vi "log analysis_gps.vi"() -> ()   [LabVIEW 2018] (continued)
normal 2 27.000000 0 0\trobot status\t-1.473744\t-2.554606\t9.902600\t-0.433320\t-1.747335\t-47.205490\t0.305000\t0.178000\n\t\n15:53:51.5\tlog_raw\tgps_raw\t#INSPVAXA,USB3,0,49.0,FINESTEERING,2107,284049.550,02008000,471d,15824;INS_ALIGNMENT_COMPLETE,INS_RTKFIXED,37.37010620824,126.72081956922,9.9012,22.3000,-0.1970,0.1771,0.0298,-0.594531132,-1.644459886,132.097505045,0.4329,0.3030,0.5941,0.1170,0.0985,0.0797,0.0945,0.0983,5.1926,0f000001,0*6b710ba0\n\tsystem status\tnormal 2 27.100000 4 0\trobot status\t-1.376142\t-2.662328\t9.901200\t-0.594531\t-1.644460\t-42.097505\t0.274000\t0.222000\n\t\n15:53:52.0\tlog_raw\tgps_raw\t#INSPVAXA,USB3,0,49.0,FINESTEERING,2107,284050.050,02008000,471d,15824;INS_ALIGNMENT_COMPLETE,INS_RTKFIXED,37.37010525413,126.72082070794,9.8986,22.3000,-0.1917,0.2051,-0.0115,-0.516834592,-1.395099600,126.953212153,0.4346,0.3025,0.5938,0.1182,0.0995,0.0796,0.0941,0.0979,5.1828,0f000001,0*22942ac6\n\tsystem status\tnormal 2 27.200000 4 0\trobot status\t-1.275276\t-2.768220\t9.898600\t-0.516835\t-1.395100\t-36.953212\t0.314000\t0.208000\n\t\n15:53:52.5\tlog_raw\tgps_raw\t#INSPVAXA,USB3,0,50.0,FINESTEERING,2107,284050.550,02008000,471d,15824;INS_ALIGNMENT_COMPLETE,INS_RTKFIXED,37.37010440811,126.72082198518,9.8945,22.3000,-0.1594,0.2362,0.0179,-0.435131967,-1.128099811,121.559655858,0.4346,0.3025,0.5938,0.1182,0.0995,0.0796,0.0941,0.0979,5.1828,0f000001,0*78d5de76\n\tsystem status\tnormal 2 27.000000 4 0\trobot status\t-1.162140\t-2.862115\t9.894500\t-0.435132\t-1.128100\t-31.559656\t0.296000\t0.194000\n\t\n15:53:53.0\tlog_raw\tgps_raw\t#DUALANTENNAHEADINGA,USB3,0,50.0,FINESTEERING,2107,284051.000,02008000,d426,15824;INSUFFICIENT_OBS,NONE,-1.000000000,0.000000000,0.000000000,0.0,0.000000000,0.000000000,\"631T\",9,3,3,3,04,00,20,00*f8ed9a8f\n\tsystem status\tnormal 2 27.100000 0 0\trobot status\t-1.053688\t-2.941976\t9.891500\t-0.278851\t-1.155266\t-26.858496\t0.311000\t0.181000\n\t\n15:53:53.5\tlog_raw\tgps_raw\t#INSPVAXA,USB3,0,49.5,FINESTEERING,2107,284051.550,02008000,471d,15824;INS_ALIGNMENT_COMPLETE,INS_RTKFIXED,37.37010293167,126.72082506603,9.8918,22.3000,-0.2006,0.4462,0.0191,-0.487315939,-0.767469623,111.533398827,0.4366,0.3027,0.5935,0.1195,0.1007,0.0795,0.0936,0.0973,5.1774,0f000001,0*2ba22a04\n\tsystem status\tnormal 2 26.900000 0 0\trobot status\t-0.889243\t-3.025977\t9.891800\t-0.487316\t-0.767470\t-21.533399\t0.466000\t0.200000\n\t\n15:53:54.0\tlog_raw\tgps_raw\t\tsystem status\tnormal 2 27.100000 4 0\trobot status\t-0.684813\t-3.109579\t9.890900\t-0.932085\t-0.917029\t-16.735766\t0.443000\t0.242000\n\t\n15:53:54.5\tlog_raw\tgps_raw\t#INSPVAXA,USB3,0,52.0,FINESTEERING,2107,284052.550,02000000,471d,15824;INS_ALIGNMENT_COMPLETE,INS_RTKFIXED,37.37010150239,126.72083015025,9.8922,22.3000,-0.0709,0.4201,0.0154,-1.300322363,-0.251250537,100.734835193,0.4385,0.3032,0.5931,0.1216,0.1015,0.0794,0.0930,0.0966,5.1757,0f000001,0*285f67bd\n\tsystem status\tnormal 2 27.000000 4 0\trobot status\t-0.438892\t-3.184605\t9.892200\t-1.300322\t-0.251251\t-10.734835\t0.551000\t0.120000\n\t\n15:53:55.0\tlog_raw\tgps_raw\t#INSPVAXA,USB3,0,51.0,FINESTEERING,2107,284053.050,02000000,471d,15824;INS_ALIGNMENT_COMPLETE,INS_RTKFIXED,37.37010109323,126.72083278272,9.8918,22.3000,-0.0521,0.4828,-0.0093,-1.553917454,-0.330463200,95.839787961,0.4397,0.3042,0.5928,0.1218,0.1030,0.0794,0.0924,0.0958,5.1723,0f000001,0*925ec3e1\n\tsystem status\tnormal 2 27.000000 4 0\trobot status\t-0.205712\t-3.230016\t9.891800\t-1.553917\t-0.330463\t-5.839788\t0.584000\t0.040000\n\t\n15:53:55.5\tlog_raw\tgps_raw\t#INSPVAXA,USB3,0,51.0,FINESTEERING,2107,284053.550,02000000,471d,15824;INS_ALIGNMENT_COMPLETE,INS_RTKFIXED,37.37010075654,126.72083555357,9.8892,22.3000,-0.0359,0.4357,0.0162,-0.976336983,-0.670873991,90.876153080,0.4397,0.3042,0.5928,0.1218,0.1030,0.0794,0.0924,0.0958,5.1723,0f000001,0*923600d8\n\tsystem status\tnormal 2 27.100000 0 0\trobot status\t0.039726\t-3.267383\t9.889200\t-0.976337\t-0.670874\t-0.876153\t0.520000\t0.127000\n\t\n15:53:56.0\tlog_raw\tgps_raw\t#INSPVAXA,USB3,0,51.0,FINESTEERING,2107,284054.050,02000000,471d,15824;INS_ALIGNMENT_COMPLETE,INS_RTKFIXED,37.37010062155,126.72083812098,9.8896,22.3000,-0.0236,0.4683,-0.0223,-0.929923548,-0.516714504,86.855289806,0.4477,0.3075,0.5936,0.1233,0.1036,0.0794,0.0919,0.0952,5.1660,0f000001,0*98660be2\n\tsystem status\tnormal 2 26.700000 4 0\trobot status\t0.267143\t-3.282365\t9.889600\t-0.929924\t-0.516715\t3.144710\t0.532000\t0.096000\n\t\n15:53:56.5\tlog_raw\tgps_raw\t#INSPVAXA,USB3,0,52.5,FINESTEERING,2107,284054.550,02000000,471d,15824;INS_ALIGNMENT_COMPLETE,INS_RTKFIXED,37.37010072634,126.72084085451,9.8879,22.3000,0.0495,0.4621,-0.0139,-0.890595687,-0.279204622,81.540293866,0.4477,0.3075,0.5936,0.1233,0.1036,0.0794,0.0919,0.0952,5.1660,0f000001,0*57c25e6b\n\tsystem status\tnormal 2 26.800000 4 0\trobot status\t0.509274\t-3.270735\t9.887900\t-0.890596\t-0.279205\t8.459706\t0.455000\t0.258000\n\t\n15:53:57.0\tlog_raw\tgps_raw\t#INSPVAXA,USB3,0,50.5,FINESTEERING,2107,284055.050,02000000,471d,15824;INS_ALIGNMENT_COMPLETE,INS_RTKFIXED,37.37010080652,126.72084262595,9.8861,22.3000,-0.0303,0.1528,0.0096,-0.789228824,0.189504141,79.603141557,0.4534,0.3102,0.5943,0.1271,0.1038,0.0794,0.0915,0.0945,5.1589,0f000001,0*17fda88b\n\tsystem status\texception 2 27.400000 4 160\trobot status\t0.666185\t-3.261836\t9.886100\t-0.789229\t0.189504\t10.396858\t0.260000\t0.206000\n\t\n15:53:57.5\tlog_raw\tgps_raw\t#INSPVAXA,USB3,0,50.5,FINESTEERING,2107,284055.550,02000000,471d,15824;INS_ALIGNMENT_COMPLETE,INS_RTKFIXED,37.37010065353,126.72084269507,9.8843,22.3000,-0.0451,0.0165,0.0094,-0.786160418,0.167323403,79.929360762,0.4534,0.3102,0.5943,0.1271,0.1038,0.0794,0.0915,0.0945,5.1589,0f000001,0*1978198f\n\tsystem status\texception 2 27.700000 0 160\trobot status\t0.672308\t-3.278816\t9.884300\t-0.786160\t0.167323\t10.070639\t0.153000\t0.216000\n\t\n15:53:58.0\tlog_raw\tgps_raw\t#INSPVAXA,USB3,0,50.5,FINESTEERING,2107,284056.050,02000000,471d,15824;INS_ALIGNMENT_COMPLETE,INS_RTKFIXED,37.37010048956,126.72084276872,9.8836,22.3000,-0.0469,0.0143,0.0092,-0.786889601,0.175933665,79.925216666,0.4574,0.3114,0.5945,0.1322,0.1037,0.0794,0.0910,0.0937,5.1545,0f000001,0*13d22f98\n\tsystem status\texception 2 27.700000 0 160\trobot status\t0.678832\t-3.297014\t9.883600\t-0.786890\t0.175934\t10.074783\t0.147000\t0.223000\n\t\n15:53:58.5\tlog_raw\tgps_raw\t#INSPVAXA,USB3,0,51.0,FINESTEERING,2107,284056.550,02000000,471d,15824;INS_ALIGNMENT_COMPLETE,INS_RTKFIXED,37.37010037074,126.72084284514,9.8838,22.3000,-0.0480,0.0175,0.0102,-0.787820604,0.175837290,79.928422775,0.4574,0.3114,0.5945,0.1322,0.1037,0.0794,0.0910,0.0937,5.1545,0f000001,0*7f57341f\n\tsystem status\texception 2 27.700000 0 160\trobot status\t0.685601\t-3.310201\t9.883800\t-0.787821\t0.175837\t10.071577\t0.147000\t0.222000\n\t\n15:53:59.0\tlog_raw\tgps_raw\t#INSPVAXA,USB3,0,51.0,FINESTEERING,2107,284057.050,02000000,471d,15824;INS_ALIGNMENT_COMPLETE,INS_RTKFIXED,37.37010024493,126.72084294147,9.8847,22.3000,-0.0489,0.0209,0.0109,-0.790474431,0.175355820,79.934854744,0.4623,0.3124,0.5946,0.1305,0.1033,0.0793,0.0905,0.0930,5.1443,0f000001,0*1624f0ca\n\tsystem status\texception 2 27.700000 0 160\trobot status\t0.694134\t-3.324164\t9.884700\t-0.790474\t0.175356\t10.065145\t0.147000\t0.222000\n\t\n15:53:59.5\tlog_raw\tgps_raw\t#INSPVAXA,USB3,0,51.0,FINESTEERING,2107,284057.550,02000000,471d,15824;INS_ALIGNMENT_COMPLETE,INS_RTKFIXED,37.37010017546,126.72084302597,9.8865,22.3000,-0.0481,0.0245,0.0114,-0.790674154,0.175795443,79.947588667,0.4623,0.3124,0.5946,0.1305,0.1033,0.0793,0.0905,0.0930,5.1443,0f000001,0*fd60ce92\n\tsystem status\texception 2 27.700000 0 160\trobot status\t0.701619\t-3.331874\t9.886500\t-0.790674\t0.175795\t10.052411\t0.147000\t0.222000\n\t\n15:54:00.0\tlog_raw\tgps_raw\t#INSPVAXA,USB3,0,51.0,FINESTEERING,2107,284058.050,02000000,471d,15824;INS_ALIGNMENT_COMPLETE,INS_RTKFIXED,37.37010009897,126.72084313411,9.8886,22.3000,-0.0478,0.0282,0.0114,-0.793625665,0.175511830,79.961034628,0.4652,0.3130,0.5946,0.1280,0.1027,0.0793,0.0901,0.0925,5.1270,0f000001,0*11f44901\n\tsystem status\tnormal 2 27.700000 0 128\trobot status\t0.711197\t-3.340363\t9.888600\t-0.793626\t0.175512\t10.038965\t0.147000\t0.222000\n\t\n15:54:00.5\tlog_raw\tgps_raw\t#INSPVAXA,USB3,0,52.5,FINESTEERING,2107,284058.550,02000000,471d,15824;INS_ALIGNMENT_COMPLETE,INS_RTKFIXED,37.37010007732,126.72084320054,9.8898,22.3000,-0.0461,0.0304,0.0122,-0.792445810,0.175564347,79.985489957,0.4652,0.3130,0.5946,0.1280,0.1027,0.0793,0.0901,0.0925,5.1270,0f000001,0*ea7ef511\n\tsystem status\texception 2 27.700000 0 160\trobot status\t0.717082\t-3.342766\t9.889800\t-0.792446\t0.175564\t10.014510\t0.147000\t0.222000\n\t\n15:54:01.0\tlog_raw\tgps_raw\t\tsystem status\texception 2 27.700000 0 160\trobot status\t0.724287\t-3.345631\t9.891600\t-0.792125\t0.176872\t9.990955\t0.147000\t0.222000\n\t\n15:54:01.5\tlog_raw\tgps_raw\t#INSPVAXA,USB3,0,48.0,FINESTEERING,2107,284059.550,02000000,471d,15824;INS_ALIGNMENT_COMPLETE,INS_RTKFIXED,37.37010006144,126.72084333190,9.8930,22.3000,-0.0410,0.0333,0.0137,-0.793411742,0.179299471,80.037482880,0.4658,0.3133,0.5945,0.1254,0.1019,0.0793,0.0898,0.0921,5.1054,0f000001,0*b41e64db\n\tsystem status\texception 2 27.700000 0 160\trobot status\t0.728717\t-3.344528\t9.893000\t-0.793412\t0.179299\t9.962517\t0.147000\t0.222000\n\t\n15:54:02.0\tlog_raw\tgps_raw\t#INSPVAXA,USB3,0,48.0,FINESTEERING,2107,284060.050,02000000,471d,15824;INS_ALIGNMENT_COMPLETE,INS_RTKFIXED,37.37010007091,126.72084339799,9.8948,22.3000,-0.0383,0.0348,0.0139,-0.792224776,0.181387989,80.068212083,0.4648,0.3132,0.5944,0.1230,0.1009,0.0793,0.0896,0.0921,5.0831,0f000001,0*0e446c66\n\tsystem status\texception 2 27.700000 0 160\trobot status\t0.734571\t-3.343477\t9.894800\t-0.792225\t0.181388\t9.931788\t0.147000\t0.222000\n\t\n15:54:02.5\tlog_raw\tgps_raw\t#INSPVAXA,USB3,0,51.5,FINESTEERING,2107,284060.550,02000000,471d,15824;INS_ALIGNMENT_COMPLETE,INS_RTKFIXED,37.37010010371,126.72084343010,9.8965,22.3000,-0.0351,0.0351,0.0141,-0.794008331,0.181387588,80.099175193,0.4648,0.3132,0.5944,0.1230,0.1009,0.0793,0.0896,0.0921,5.0831,0f000001,0*6d5ef346\n\tsystem status\texception 2 27.700000 0 160\trobot status\t0.737416\t-3.339837\t9.896500\t-0.794008\t0.181388\t9.900825\t0.147000\t0.222000\n\t\n15:54:03.0\tlog_raw\tgps_raw\t#INSPVAXA,USB3,0,47.0,FINESTEERING,2107,284061.050,02000000,471d,15824;INS_ALIGNMENT_COMPLETE,INS_RTKFIXED,37.37010013657,126.72084347859,9.8982,22.3000,-0.0318,0.0362,0.0140,-0.793134778,0.182296813,80.130371651,0.4625,0.3128,0.5942,0.1207,0.0997,0.0793,0.0895,0.0922,5.0625,0f000001,0*150e9f64\n\tsystem status\texception 2 27.700000 0 160\trobot status\t0.741711\t-3.336190\t9.898200\t-0.793135\t0.182297\t9.869628\t0.147000\t0.222000\n\t\n15:54:03.5\tlog_raw\tgps_raw\t\tsystem status\texception 2 27.700000 0 160\trobot status\t0.745103\t-3.333746\t9.898900\t-0.794686\t0.183659\t9.841140\t0.147000\t0.222000\n\t\n15:54:04.0\tlog_raw\tgps_raw\t#INSPVAXA,USB3,0,47.0,FINESTEERING,2107,284062.050,02000000,471d,15824;INS_ALIGNMENT_COMPLETE,INS_RTKFIXED,37.37010017748,126.72084356719,9.8997,22.3000,-0.0290,0.0363,0.0139,-0.794331592,0.183823168,80.187481896,0.4594,0.3121,0.5941,0.1189,0.0986,0.0793,0.0895,0.0925,5.0451,0f000001,0*0cfca1c0\n\tsystem status\texception 2 27.800000 0 160\trobot status\t0.749559\t-3.331650\t9.899700\t-0.794332\t0.183823\t9.812518\t0.147000\t0.222000\n\t\n15:54:04.5\tlog_raw\tgps_raw\t\tsystem status\texception 2 27.700000 0 160\trobot status\t0.750935\t-3.327984\t9.900000\t-0.792965\t0.186753\t9.783400\t0.147000\t0.222000\n\t\n15:54:05.0\tlog_raw\tgps_raw\t#INSPVAXA,USB3,0,47.5,FINESTEERING,2107,284063.050,02000000,471d,15824;INS_ALIGNMENT_COMPLETE,INS_RTKFIXED,37.37010026095,126.72084358162,9.8989,22.3000,-0.0250,0.0360,0.0144,-0.793980547,0.188879000,80.251853132,0.3252,0.2278,0.4744,0.0459,0.0444,0.0422,0.0723,0.0737,4.9906,0f000005,0*164f8940\n\tsystem status\tnormal 2 27.800000 0 128\trobot status\t0.750837\t-3.322386\t9.898900\t-0.793981\t0.188879\t9.748147\t0.147000\t0.222000\n\t\n15:54:05.5\tlog_raw\tgps_raw\t#INSPVAXA,USB3,0,47.5,FINESTEERING,2107,284063.550,02000000,471d,15824;INS_ALIGNMENT_COMPLETE,INS_RTKFIXED,37.37010060191,126.72084312304,9.8728,22.3000,-0.0145,0.0225,0.0107,-0.798483661,0.197892830,80.372723663,0.3252,0.2278,0.4744,0.0459,0.0444,0.0422,0.0723,0.0737,4.9906,0f000005,0*92bf4382\n\tsystem status\texception 2 27.700000 0 160\trobot status\t0.710217\t-3.284545\t9.872800\t-0.798484\t0.197893\t9.627276\t0.147000\t0.222000\n\t\n15:54:06.0\tlog_raw\tgps_raw\t#INSPVAXA,USB3,0,47.5,FINESTEERING,2107,284064.050,02000000,471d,15824;INS_ALIGNMENT_COMPLETE,INS_RTKFIXED,37.37010092341,126.72084268927,9.8479,22.3000,-0.0050,0.0083,0.0065,-0.802010918,0.203072267,80.489552578,0.3043,0.2119,0.4435,0.0375,0.0370,0.0348,0.0717,0.0735,4.9827,0f000005,0*2a9229fa\n\tsystem status\texception 2 27.700000 0 160\trobot status\t0.671794\t-3.248863\t9.847900\t-0.802011\t0.203072\t9.510447\t0.147000\t0.222000\n\t\n15:54:06.5\tlog_raw\tgps_raw\t#INSPVAXA,USB3,0,52.0,FINESTEERING,2107,284064.550,02000000,471d,15824;INS_ALIGNMENT_COMPLETE,INS_RTKFIXED,37.37010093886,126.72084266042,9.8416,22.3000,-0.0043,0.0064,0.0059,-0.803970150,0.202555305,80.508100729,0.3043,0.2119,0.4435,0.0375,0.0370,0.0348,0.0717,0.0735,4.9827,0f000005,0*b303c02a\n\tsystem status\texception 2 27.800000 0 160\trobot status\t0.669239\t-3.247148\t9.841600\t-0.803970\t0.202555\t9.491899\t0.147000\t0.222000\n\t\n15:54:07.0\tlog_raw\tgps_raw\t#INSPVAXA,USB3,0,48.0,FINESTEERING,2107,284065.050,02000000,471d,15824;INS_ALIGNMENT_COMPLETE,INS_RTKFIXED,37.37010095172,126.72084263427,9.8359,22.3000,-0.0031,0.0050,0.0058,-0.803101201,0.203067002,80.525514277,0.2907,0.2017,0.4242,0.0352,0.0350,0.0325,0.0719,0.0737,4.9778,0f000005,0*fc85e648\n\tsystem status\tnormal 2 27.800000 0 128\trobot status\t0.666922\t-3.245721\t9.835900\t-0.803101\t0.203067\t9.474486\t0.147000\t0.222000\n\t\n15:54:07.5\tlog_raw\tgps_raw\t\tsystem status\texception 2 27.700000 0 160\trobot status\t0.667591\t-3.245814\t9.833800\t-0.802684\t0.201518\t9.473939\t0.147000\t0.222000\n\t\n15:54:08.0\tlog_raw\tgps_raw\t\tsystem status\texception 0 27.700000 0 32\trobot status\t0.668973\t-3.245733\t9.832100\t-0.803936\t0.200249\t9.474753\t0.147000\t0.222000\n\t\n15:54:08.5\tlog_raw\tgps_raw\t#INSPVAXA,USB3,0,50.0,FINESTEERING,2107,284066.550,02000000,471d,15824;INS_ALIGNMENT_COMPLETE,INS_RTKFIXED,37.37010094761,126.72084266483,9.8311,22.3000,-0.0007,0.0064,0.0053,-0.805322808,0.199332071,80.524990625,0.2793,0.1938,0.4090,0.0347,0.0344,0.0317,0.0721,0.0737,4.9673,0f000005,0*f499bec4\n\tsystem status\texception 0 27.800000 0 32\trobot status\t0.669629\t-3.246177\t9.831100\t-0.805323\t0.199332\t9.475009\t0.147000\t0.222000\n\t\n15:54:09.0\tlog_raw\tgps_raw\t#INSPVAXA,USB3,0,45.0,FINESTEERING,2107,284067.050,02000000,471d,15824;INS_ALIGNMENT_COMPLETE,INS_RTKFIXED,37.37010094387,126.72084267852,9.8307,22.3000,-0.0007,0.0065,0.0059,-0.804077571,0.201412948,80.525848539,0.2693,0.1873,0.3960,0.0346,0.0343,0.0314,0.0722,0.0736,4.9532,0f000005,0*b106a646\n\tsystem status\texception 0 27.800000 0 32\trobot status\t0.670842\t-3.246592\t9.830700\t-0.804078\t0.201413\t9.474151\t0.147000\t0.222000\n\t\n15:54:09.5\tlog_raw\tgps_raw\t\tsystem status\texception 0 27.800000 0 32\trobot status\t0.671565\t-3.247256\t9.830100\t-0.803361\t0.201716\t9.474638\t0.147000\t0.222000\n\t\n15:54:10.0\tlog_raw\tgps_raw\t#INSPVAXA,USB3,0,45.0,FINESTEERING,2107,284068.050,02000000,471d,15824;INS_ALIGNMENT_COMPLETE,INS_RTKFIXED,37.37010093147,126.72084269859,9.8300,22.3000,-0.0011,0.0054,0.0061,-0.802134558,0.201672823,80.524962469,0.2605,0.1821,0.3846,0.0346,0.0343,0.0313,0.0723,0.0734,4.9387,0f000005,0*023ab06f\n\tsystem status\texception 0 27.800000 0 32\trobot status\t0.672620\t-3.247969\t9.830000\t-0.802135\t0.201673\t9.475038\t0.147000\t0.222000\n\t\n15:54:10.5\tlog_raw\tgps_raw\t\tsystem status\texception 0 27.800000 0 32\trobot status\t0.673184\t-3.248426\t9.829300\t-0.800656\t0.202458\t9.475344\t0.147000\t0.222000\n\t\n15:54:11.0\tlog_raw\tgps_raw\t\tsystem status\texception 0 27.800000 0 32\trobot status\t0.674167\t-3.248973\t9.829300\t-0.799789\t0.203840\t9.478232\t0.147000\t0.222000\n\t\n15:54:11.5\tlog_raw\tgps_raw\t#INSPVAXA,USB3,0,52.5,FINESTEERING,2107,284069.550,02000000,471d,15824;INS_ALIGNMENT_COMPLETE,INS_RTKFIXED,37.37010092244,126.72084272464,9.8293,22.3000,-0.0013,0.0057,0.0059,-0.798598974,0.203976276,80.516419675,0.2537,0.1782,0.3747,0.0345,0.0343,0.0313,0.0723,0.0733,4.9257,0f000005,0*56198093\n\tsystem status\texception 0 27.700000 0 32\trobot status\t0.674927\t-3.248971\t9.829300\t-0.798599\t0.203976\t9.483580\t0.147000\t0.222000\n\t\n15:54:12.0\tlog_raw\tgps_raw\t#INSPVAXA,USB3,0,52.5,FINESTEERING,2107,284070.050,02000000,471d,15824;INS_ALIGNMENT_COMPLETE,INS_RTKFIXED,37.37010091982,126.72084273744,9.8297,22.3000,-0.0012,0.0080,0.0052,-0.796727291,0.202371402,80.509450854,0.2478,0.1752,0.3659,0.0345,0.0343,0.0313,0.0724,0.0732,4.9128,0f000005,0*32eb7788\n\tsystem status\texception 0 27.800000 0 32\trobot status\t0.676061\t-3.249262\t9.829700\t-0.796727\t0.202371\t9.490549\t0.147000\t0.222000\n\t\n15:54:12.5\tlog_raw\tgps_raw\t\tsystem status\texception 0 27.800000 0 32\trobot status\t0.674655\t-3.249824\t9.829400\t-0.792783\t0.205130\t9.497173\t0.147000\t0.222000\n\t\n15:54:13.0\tlog_raw\tgps_raw\t#INSPVAXA,USB3,0,48.5,FINESTEERING,2107,284071.050,02000000,471d,15824;INS_ALIGNMENT_COMPLETE,INS_RTKFIXED,37.37010090434,126.72084271110,9.8295,22.3000,-0.0039,0.0026,0.0058,-0.794464008,0.206738241,80.502187928,0.2427,0.1727,0.3579,0.0345,0.0343,0.0313,0.0724,0.0732,4.9038,0f000005,0*ae7eb45b\n\tsystem status\texception 0 27.800000 0 32\trobot status\t0.673728\t-3.250980\t9.829500\t-0.794464\t0.206738\t9.497812\t0.147000\t0.222000\n\t\n15:54:13.5\tlog_raw\tgps_raw\t#INSPVAXA,USB3,0,48.5,FINESTEERING,2107,284071.550,02000000,471d,15824;INS_ALIGNMENT_COMPLETE,INS_RTKFIXED,37.37010089734,126.72084271003,9.8294,22.3000,-0.0047,0.0026,0.0048,-0.792309552,0.204330401,80.495522274,0.2427,0.1727,0.3579,0.0345,0.0343,0.0313,0.0724,0.0732,4.9038,0f000005,0*ad98db8e\n\tsystem status\texception 0 27.800000 0 32\trobot status\t0.673633\t-3.251756\t9.829400\t-0.792310\t0.204330\t9.504478\t0.147000\t0.222000\n\t\n15:54:14.0\tlog_raw\tgps_raw\t\tsystem status\texception 0 27.800000 0 32\trobot status\t0.673376\t-3.253810\t9.829800\t-0.795967\t0.184821\t9.359598\t0.117000\t0.095000\n\t\n15:54:14.5\tlog_raw\tgps_raw\t\tsystem status\texception 0 27.800000 0 60\trobot status\t0.674132\t-3.257605\t9.832900\t-0.788414\t0.193198\t9.387077\t0.117000\t0.095000\n\t\n15:54:15.0\tlog_raw\tgps_raw\t\tsystem status\texception 0 27.800000 0 60\trobot status\t0.676499\t-3.262353\t9.836500\t-0.786147\t0.194904\t9.385323\t0.117000\t0.095000\n\t\n15:54:15.5\tlog_raw\tgps_raw\t\tsystem status\texception 0 27.800000 0 60\trobot status\t0.678961\t-3.267673\t9.840700\t-0.786580\t0.194426\t9.385900\t0.117000\t0.095000\n\t\n15:54:16.0\tlog_raw\tgps_raw\t\tsystem status\texception 0 27.800000 0 60\trobot status\t0.682045\t-3.274174\t9.845300\t-0.785139\t0.194086\t9.384595\t0.117000\t0.095000\n\t\n15:54:16.5\tlog_raw\tgps_raw\t\tsystem status\texception 0 27.800000 0 60\trobot status\t0.684298\t-3.281012\t9.849500\t-0.785110\t0.192293\t9.376254\t0.117000\t0.095000\n\t\n15:54:17.0\tlog_raw\tgps_raw\t\tsystem status\texception 0 27.800000 0 60\trobot status\t0.687811\t-3.288802\t9.854200\t-0.783660\t0.192337\t9.377009\t0.117000\t0.095000\n\t\n15:54:17.5\tlog_raw\tgps_raw\t\tsystem status\texception 0 27.800000 0 60\trobot status\t0.690737\t-3.295775\t9.858800\t-0.784560\t0.190680\t9.377608\t0.117000\t0.095000\n\t\n15:54:18.0\tlog_raw\tgps_raw\t#INSPVAXA,USB3,0,53.5,FINESTEERING,2107,284076.050,02000000,471d,15824;INS_ALIGNMENT_COMPLETE,INS_RTKFIXED,37.37010043153,126.72084293702,9.8639,22.3000,-0.0224,0.0084,0.0124,-0.782520442,0.190697298,80.620510756,0.3079,0.2467,0.3912,0.0928,0.0849,0.0629,0.0895,0.0915,4.9091,0f000001,0*151fdb37\n\tsystem status\texception 0 27.800000 0 60\trobot status\t0.693740\t-3.303454\t9.863900\t-0.782520\t0.190697\t9.379489\t0.117000\t0.095000\n\t\n15:54:18.5\tlog_raw\tgps_raw\t\tsystem status\texception 0 27.800000 0 60\trobot status\t0.697678\t-3.308999\t9.869500\t-0.783353\t0.190598\t9.384457\t0.117000\t0.095000\n\t\n15:54:19.0\tlog_raw\tgps_raw\t\tsystem status\texception 0 27.800000 0 60\trobot status\t0.701548\t-3.315091\t9.875400\t-0.783389\t0.191366\t9.388017\t0.117000\t0.095000\n\t\n15:54:19.5\tlog_raw\tgps_raw\t#INSPVAXA,USB3,0,53.0,FINESTEERING,2107,284077.550,02000000,471d,15824;INS_ALIGNMENT_COMPLETE,INS_RTKFIXED,37.37010029205,126.72084303769,9.8807,22.3000,-0.0245,0.0085,0.0134,-0.783196665,0.189878552,80.605229248,0.3387,0.2662,0.4111,0.1003,0.0889,0.0668,0.0907,0.0935,4.9083,0f000001,0*a805bdc6\n\tsystem status\texception 0 27.800000 0 60\trobot status\t0.702657\t-3.318934\t9.880700\t-0.783197\t0.189879\t9.394771\t0.117000\t0.095000\n\t\n15:54:20.0\tlog_raw\tgps_raw\t\tsystem status\tnormal 0 27.800000 0 0\trobot status\t0.703458\t-3.323399\t9.886200\t-0.780694\t0.190160\t9.399105\t0.000000\t0.000000\n\t\n15:54:20.5\tlog_raw\tgps_raw\t\tsystem status\tnormal 0 27.800000 0 0\trobot status\t0.702893\t-3.324862\t9.890500\t-0.780697\t0.189721\t9.404535\t0.000000\t0.000000\n\t\n15:54:21.0\tlog_raw\tgps_raw\t\tsystem status\tnormal 0 27.800000 0 0\trobot status\t0.702016\t-3.324874\t9.893500\t-0.780007\t0.186169\t9.412956\t0.000000\t0.000000\n\t\n15:54:21.5\tlog_raw\tgps_raw\t\tsystem status\tnormal 0 27.800000 0 0\trobot status\t0.692362\t-3.293473\t9.874500\t-0.787467\t0.184565\t9.458727\t0.000000\t0.000000\n\t\n15:54:22.0\tlog_raw\tgps_raw\t\tsystem status\tnormal 0 27.800000 0 0\trobot status\t0.683376\t-3.263954\t9.856300\t-0.789770\t0.183627\t9.504189\t0.000000\t0.000000\n\t\n15:54:22.5\tlog_raw\tgps_raw\t\tsystem status\tnormal 0 27.800000 0 0\trobot status\t0.682030\t-3.260340\t9.853100\t-0.787874\t0.181330\t9.515919\t0.000000\t0.000000\n\t\n15:54:23.0\tlog_raw\tgps_raw\t\tsystem status\tnormal 0 27.800000 0 0\trobot status\t0.681223\t-3.257523\t9.850000\t-0.789565\t0.179310\t9.527684\t0.000000\t0.000000\n\t\n15:54:23.5\tlog_raw\tgps_raw\t\tsystem status\tnormal 0 27.800000 0 0\trobot status\t0.680455\t-3.255804\t9.848800\t-0.790395\t0.180071\t9.535480\t0.000000\t0.000000\n\t\n15:54:24.0\tlog_raw\tgps_raw\t\tsystem status\tnormal 0 27.800000 0 0\trobot status\t0.680334\t-3.254433\t9.847700\t-0.791047\t0.181331\t9.542257\t0.000000\t0.000000\n\t\n15:54:24.5\tlog_raw\tgps_raw\t\tsystem status\tnormal 0 27.800000 0 0\trobot status\t0.680342\t-3.253833\t9.847500\t-0.791894\t0.181200\t9.547376\t0.000000\t0.000000\n\t\n15:54:25.0\tlog_raw\tgps_raw\t\tsystem status\tnormal 0 27.800000 0 0\trobot status\t0.680929\t-3.253774\t9.847400\t-0.791843\t0.181231\t9.550330\t0.000000\t0.000000\n\t\n15:54:25.5\tlog_raw\tgps_raw\t\tsystem status\tnormal 0 27.800000 0 0\trobot status\t0.681186\t-3.253691\t9.847000\t-0.789831\t0.179723\t9.554560\t0.000000\t0.000000\n\t\n15:54:26.0\tlog_raw\tgps_raw\t\tsystem status\tnormal 0 27.800000 0 0\trobot status\t0.682117\t-3.254210\t9.846700\t-0.790189\t0.179013\t9.555721\t0.000000\t0.000000\n\t\n15:54:26.6\tlog_raw\tgps_raw\t\tsystem status\tnormal 0 27.800000 0 0\trobot status\t0.681923\t-3.253710\t9.846600\t-0.791346\t0.177690\t9.559489\t0.000000\t0.000000\n\t\n15:54:27.1\tlog_raw\tgps_raw\t\tsystem status\tnormal 0 27.800000 0 0\trobot status\t0.682013\t-3.253657\t9.846600\t-0.793372\t0.178535\t9.563909\t0.000000\t0.000000\n\t\n15:54:27.6\tlog_raw\tgps_raw\t\tsystem status\tnormal 0 27.800000 0 0\trobot status\t0.681908\t-3.253389\t9.846400\t-0.792445\t0.179401\t9.567671\t0.000000\t0.000000\n\t\n15:54:28.1\tlog_raw\tgps_raw\t\tsystem status\tnormal 0 27.800000 0 0\trobot status\t0.682395\t-3.253468\t9.846300\t-0.794347\t0.178759\t9.573326\t0.000000\t0.000000\n\t\n15:54:28.6\tlog_raw\tgps_raw\t\tsystem status\tnormal 0 27.800000 0 0\trobot status\t0.682458\t-3.252987\t9.846100\t-0.793175\t0.179425\t9.576746\t0.000000\t0.000000\n\t\n15:54:29.1\tlog_raw\tgps_raw\t\tsystem status\tnormal 0 27.800000 0 0\trobot status\t0.683140\t-3.252620\t9.846200\t-0.794003\t0.178881\t9.582150\t0.000000\t0.000000\n\t\n15:54:29.6\tlog_raw\tgps_raw\t\tsystem status\tnormal 0 27.800000 0 0\trobot status\t0.683415\t-3.252631\t9.846200\t-0.793579\t0.179588\t9.585333\t0.000000\t0.000000\n\t\n15:54:30.1\tlog_raw\tgps_raw\t\tsystem status\tnormal 0 27.800000 0 0\trobot status\t0.684398\t-3.253129\t9.846700\t-0.790496\t0.179552\t9.586305\t0.000000\t0.000000\n\t\n15:54:30.6\tlog_raw\tgps_raw\t\tsystem status\tnormal 0 27.800000 0 0\trobot status\t0.684170\t-3.252896\t9.846100\t-0.789948\t0.181891\t9.589543\t0.000000\t0.000000\n\t\n15:54:31.1\tlog_raw\tgps_raw\t\tsystem status\tnormal 0 27.800000 0 0\trobot status\t0.684077\t-3.253163\t9.845600\t-0.788367\t0.183688\t9.593241\t0.000000\t0.000000\n\t\n15:54:31.6\tlog_raw\tgps_raw\t\tsystem status\tnormal 0 27.800000 0 0\trobot status\t0.683681\t-3.252744\t9.844800\t-0.787114\t0.186011\t9.597892\t0.000000\t0.000000\n\t\n15:54:32.1\tlog_raw\tgps_raw\t\tsystem status\tnormal 0 27.800000 0 0\trobot status\t0.683322\t-3.252677\t9.843800\t-0.785050\t0.188708\t9.600820\t0.000000\t0.000000\n\t\n15:54:32.6\tlog_raw\tgps_raw\t\tsystem status\tnormal 0 27.800000 0 0\trobot status\t0.682764\t-3.252590\t9.843200\t-0.782479\t0.192998\t9.604699\t0.000000\t0.000000\n\t\n15:54:33.1\tlog_raw\tgps_raw\t\tsystem status\tnormal 0 27.800000 0 0\trobot status\t0.682458\t-3.253261\t9.842400\t-0.780713\t0.192499\t9.605498\t0.000000\t0.000000\n\t\n15:54:33.6\tlog_raw\tgps_raw\t\tsystem status\tnormal 0 27.800000 0 0\trobot status\t0.682185\t-3.253004\t9.841900\t-0.779613\t0.191968\t9.608603\t0.000000\t0.000000\n\t\n15:54:34.1\tlog_raw\tgps_raw\t\tsystem status\tnormal 0 27.800000 0 0\trobot status\t0.682287\t-3.253367\t9.841400\t-0.778829\t0.193122\t9.609729\t0.000000\t0.000000\n\t\n15:54:34.6\tlog_raw\tgps_raw\t\tsystem status\tnormal 0 27.800000 0 0\trobot status\t0.681749\t-3.253302\t9.840700\t-0.778825\t0.193112\t9.612888\t0.000000\t0.000000\n\t\n15:54:35.1\tlog_raw\tgps_raw\t\tsystem status\tnormal 0 27.800000 0 0\trobot status\t0.681854\t-3.254215\t9.840500\t-0.778716\t0.195245\t9.615071\t0.000000\t0.000000\n\t\n15:54:35.6\tlog_raw\tgps_raw\t\tsystem status\tnormal 0 27.800000 0 0\trobot status\t0.681488\t-3.254019\t9.840300\t-0.777265\t0.194342\t9.619581\t0.000000\t0.000000\n\t\n15:54:36.1\tlog_raw\tgps_raw\t\tsystem status\tnormal 0 27.800000 0 0\trobot status\t0.681478\t-3.254648\t9.840500\t-0.777409\t0.195182\t9.625489\t0.000000\t0.000000\n\t\n15:54:36.6\tlog_raw\tgps_raw\t\tsystem status\tnormal 0 27.800000 0 0\trobot status\t0.681376\t-3.254824\t9.840000\t-0.777101\t0.196484\t9.630293\t0.000000\t0.000000\n\t\n15:54:37.1\tlog_raw\tgps_raw\t\tsystem status\tnormal 0 27.800000 0 0\trobot status\t0.681842\t-3.256278\t9.839600\t-0.777886\t0.194547\t9.634677\t0.000000\t0.000000\n\t\n15:54:37.6\tlog_raw\tgps_raw\t\tsystem status\tnormal 0 27.800000 0 0\trobot status\t0.681971\t-3.256801\t9.839500\t-0.777016\t0.195175\t9.639378\t0.000000\t0.000000\n\t\n15:54:38.1\tlog_raw\tgps_raw\t\tsystem status\tnormal 0 27.800000 0 0\trobot status\t0.682875\t-3.258832\t9.839600\t-0.778246\t0.195711\t9.645257\t0.000000\t0.000000\n\t\n15:54:38.6\tlog_raw\tgps_raw\t\tsystem status\tnormal 0 27.800000 0 0\trobot status\t0.682641\t-3.258653\t9.839600\t-0.776747\t0.198065\t9.652913\t0.000000\t0.000000\n\t\n15:54:39.1\tlog_raw\tgps_raw\t\tsystem status\tnormal 0 27.800000 0 0\trobot status\t0.682671\t-3.259591\t9.839700\t-0.776372\t0.199339\t9.658868\t0.000000\t0.000000\n\t\n15:54:39.6\tlog_raw\tgps_raw\t\tsystem status\tnormal 0 27.800000 0 0\trobot status\t0.682346\t-3.259470\t9.839500\t-0.776737\t0.200947\t9.667602\t0.000000\t0.000000\n\t\n15:54:40.1\tlog_raw\tgps_raw\t#INSPVAXA,USB3,0,52.0,FINESTEERING,2107,284098.100,02000000,471d,15824;INS_ALIGNMENT_COMPLETE,INS_RTKFIXED,37.37010081715,126.72084280567,9.8392,22.3000,-0.0127,0.0026,0.0011,-0.779185291,0.204850370,80.324830339,0.2135,0.1621,0.2919,0.0344,0.0343,0.0312,0.0727,0.0733,4.8847,0f000005,0*b965a086\n\tsystem status\tnormal 0 27.800000 0 0\trobot status\t0.682105\t-3.260656\t9.839200\t-0.779185\t0.204850\t9.675170\t0.000000\t0.000000\n\t\n15:54:40.6\tlog_raw\tgps_raw\t\tsystem status\tnormal 0 27.800000 0 0\trobot status\t0.682081\t-3.260836\t9.839000\t-0.778025\t0.205911\t9.681389\t0.000000\t0.000000\n\t\n15:54:41.1\tlog_raw\tgps_raw\t#INSPVAXA,USB3,0,53.0,FINESTEERING,2107,284099.100,02000000,471d,15824;INS_ALIGNMENT_COMPLETE,INS_RTKFIXED,37.37010080039,126.72084280580,9.8388,22.3000,-0.0144,0.0013,0.0007,-0.778559962,0.207012458,80.310324133,0.2130,0.1619,0.2904,0.0344,0.0343,0.0312,0.0727,0.0733,4.8855,0f000005,0*91b9a8e7\n\tsystem status\tnormal 0 27.800000 0 0\trobot status\t0.682116\t-3.262516\t9.838800\t-0.778560\t0.207012\t9.689676\t0.000000\t0.000000\n\t\n15:54:41.6\tlog_raw\tgps_raw\t\tsystem status\tnormal 0 27.800000 0 0\trobot status\t0.681851\t-3.262232\t9.838600\t-0.780123\t0.208991\t9.696795\t0.000000\t0.000000\n\t\n15:54:42.1\tlog_raw\tgps_raw\t\tsystem status\tnormal 0 27.800000 0 0\trobot status\t0.681423\t-3.262914\t9.838200\t-0.782128\t0.209689\t9.702959\t0.000000\t0.000000\n\t\n15:54:42.6\tlog_raw\tgps_raw\t\tsystem status\tnormal 0 27.800000 0 0\trobot status\t0.681331\t-3.262336\t9.837800\t-0.783864\t0.208964\t9.709043\t0.000000\t0.000000\n\t\n15:54:43.1\tlog_raw\tgps_raw\t#INSPVAXA,USB3,0,50.0,FINESTEERING,2107,284101.100,02000000,471d,15824;INS_ALIGNMENT_COMPLETE,INS_RTKFIXED,37.37010080256,126.72084279427,9.8376,22.3000,-0.0100,0.0003,0.0004,-0.784971071,0.210053203,80.284000785,0.2120,0.1618,0.2876,0.0344,0.0343,0.0312,0.0727,0.0733,4.8873,0f000005,0*ce207b7d\n\tsystem status\tnormal 0 27.800000 0 0\trobot status\t0.681095\t-3.262276\t9.837600\t-0.784971\t0.210053\t9.715999\t0.000000\t0.000000\n\t\n15:54:43.6\tlog_raw\tgps_raw\t#INSPVAXA,USB3,0,50.0,FINESTEERING,2107,284101.600,02000000,471d,15824;INS_ALIGNMENT_COMPLETE,INS_RTKFIXED,37.37010080771,126.72084279588,9.8375,22.3000,-0.0097,0.0008,0.0002,-0.787245577,0.212021074,80.277840242,0.2120,0.1618,0.2876,0.0344,0.0343,0.0312,0.0727,0.0733,4.8873,0f000005,0*d3394abe\n\tsystem status\tnormal 0 27.800000 0 0\trobot status\t0.681238\t-3.261704\t9.837500\t-0.787246\t0.212021\t9.722160\t0.000000\t0.000000\n\t\n15:54:44.1\tlog_raw\tgps_raw\t#INSPVAXA,USB3,0,53.0,FINESTEERING,2107,284102.100,02000000,471d,15824;INS_ALIGNMENT_COMPLETE,INS_RTKFIXED,37.37010080827,126.72084279791,9.8372,22.3000,-0.0086,0.0007,-0.0005,-0.787222200,0.211318071,80.272885297,0.2116,0.1617,0.2864,0.0344,0.0343,0.0312,0.0727,0.0733,4.8883,0f000005,0*7e8ab6e8\n\tsystem status\tnormal 0 27.800000 0 0\trobot status\t0.681417\t-3.261642\t9.837200\t-0.787222\t0.211318\t9.727115\t0.000000\t0.000000\n\t\n15:54:44.6\tlog_raw\tgps_raw\t\tsystem status\tnormal 0 27.800000 0 0\trobot status\t0.681052\t-3.260775\t9.836800\t-0.788225\t0.213463\t9.733143\t0.000000\t0.000000\n\t\n15:54:45.1\tlog_raw\tgps_raw\t#INSPVAXA,USB3,0,53.0,FINESTEERING,2107,284103.100,02000000,471d,15824;INS_ALIGNMENT_COMPLETE,INS_RTKFIXED,37.37010082403,126.72084278484,9.8365,22.3000,-0.0064,-0.0008,-0.0001,-0.787428816,0.215864037,80.263823554,0.2112,0.1616,0.2853,0.0344,0.0343,0.0312,0.0727,0.0733,4.8894,0f000005,0*f475c441\n\tsystem status\tnormal 0 27.800000 0 0\trobot status\t0.680260\t-3.259893\t9.836500\t-0.787429\t0.215864\t9.736176\t0.000000\t0.000000\n\t\n15:54:45.6\tlog_raw\tgps_raw\t\tsystem status\tnormal 0 27.800000 0 0\trobot status\t0.680156\t-3.259534\t9.836400\t-0.785990\t0.217629\t9.740440\t0.000000\t0.000000\n\t\n15:54:46.1\tlog_raw\tgps_raw\t#INSPVAXA,USB3,0,53.0,FINESTEERING,2107,284104.050,02000000,471d,15824;INS_ALIGNMENT_COMPLETE,INS_RTKFIXED,37.37010082408,126.72084278410,9.8363,22.3000,-0.0077,0.0002,0.0002,-0.786930858,0.220983047,80.255496235,0.2109,0.1616,0.2842,0.0344,0.0343,0.0312,0.0727,0.0733,4.8905,0f000005,0*84218c18\n\tsystem status\tnormal 0 27.800000 0 0\trobot status\t0.680194\t-3.259887\t9.836300\t-0.786931\t0.220983\t9.744504\t0.000000\t0.000000\n\t\n15:54:46.6\tlog_raw\tgps_raw\t#INSPVAXA,USB3,0,53.0,FINESTEERING,2107,284104.050,02000000,471d,15824;INS_ALIGNMENT_COMPLETE,INS_RTKFIXED,37.37010082408,126.72084278410,9.8363,22.3000,-0.0077,0.0002,0.0002,-0.786930858,0.220983047,80.255496235,0.2109,0.1616,0.2842,0.0344,0.0343,0.0312,0.0727,0.0733,4.8905,0f000005,0*84218c18\n\tsystem status\tnormal 0 27.800000 0 0\trobot status\t0.680194\t-3.259887\t9.836300\t-0.786931\t0.220983\t9.744504\t0.000000\t0.000000\n\t\n15:54:47.1\tlog_raw\tgps_raw\t#INSPVAXA,USB3,0,53.0,FINESTEERING,2107,284104.050,02000000,471d,15824;INS_ALIGNMENT_COMPLETE,INS_RTKFIXED,37.37010082408,126.72084278410,9.8363,22.3000,-0.0077,0.0002,0.0002,-0.786930858,0.220983047,80.255496235,0.2109,0.1616,0.2842,0.0344,0.0343,0.0312,0.0727,0.0733,4.8905,0f000005,0*84218c18\n\tsystem status\tnormal 0 27.800000 0 0\trobot status\t0.680194\t-3.259887\t9.836300\t-0.786931\t0.220983\t9.744504\t0.000000\t0.000000\n\t\n15:54:47.6\tlog_raw\tgps_raw\t#INSPVAXA,USB3,0,53.0,FINESTEERING,2107,284104.050,02000000,471d,15824;INS_ALIGNMENT_COMPLETE,INS_RTKFIXED,37.37010082408,126.72084278410,9.8363,22.3000,-0.0077,0.0002,0.0002,-0.786930858,0.220983047,80.255496235,0.2109,0.1616,0.2842,0.0344,0.0343,0.0312,0.0727,0.0733,4.8905,0f000005,0*84218c18\n\tsystem status\tnormal 0 27.800000 0 0\trobot status\t0.680194\t-3.259887\t9.836300\t-0.786931\t0.220983\t9.744504\t0.000000\t0.000000\n\t\n15:54:48.1\tlog_raw\tgps_raw\t#INSPVAXA,USB3,0,53.0,FINESTEERING,2107,284104.050,02000000,471d,15824;INS_ALIGNMENT_COMPLETE,INS_RTKFIXED,37.37010082408,126.72084278410,9.8363,22.3000,-0.0077,0.0002,0.0002,-0.786930858,0.220983047,80.255496235,0.2109,0.1616,0.2842,0.0344,0.0343,0.0312,0.0727,0.0733,4.8905,0f000005,0*84218c18\n\tsystem status\tnormal 0 27.800000 0 0\trobot status\t0.680194\t-3.259887\t9.836300\t-0.786931\t0.220983\t9.744504\t0.000000\t0.000000\n\t\n15:54:48.6\tlog_raw\tgps_raw\t#INSPVAXA,USB3,0,53.0,FINESTEERING,2107,284104.050,02000000,471d,15824;INS_ALIGNMENT_COMPLETE,INS_RTKFIXED,37.37010082408,126.72084278410,9.8363,22.3000,-0.0077,0.0002,0.0002,-0.786930858,0.220983047,80.255496235,0.2109,0.1616,0.2842,0.0344,0.0343,0.0312,0.0727,0.0733,4.8905,0f000005,0*84218c18\n\tsystem status\tnormal 0 27.800000 0 0\trobot status\t0.680194\t-3.259887\t9.836300\t-0.786931\t0.220983\t9.744504\t0.000000\t0.000000\n\t\n15:54:49.1\tlog_raw\tgps_raw\t#INSPVAXA,USB3,0,53.0,FINESTEERING,2107,284104.050,02000000,471d,15824;INS_ALIGNMENT_COMPLETE,INS_RTKFIXED,37.37010082408,126.72084278410,9.8363,22.3000,-0.0077,0.0002,0.0002,-0.786930858,0.220983047,80.255496235,0.2109,0.1616,0.2842,0.0344,0.0343,0.0312,0.0727,0.0733,4.8905,0f000005,0*84218c18\n\tsystem status\tnormal 0 27.800000 0 0\trobot status\t0.680194\t-3.259887\t9.836300\t-0.786931\t0.220983\t9.744504\t0.000000\t0.000000\n\t\n15:54:49.6\tlog_raw\tgps_raw\t#INSPVAXA,USB3,0,53.0,FINESTEERING,2107,284104.050,02000000,471d,15824;INS_ALIGNMENT_COMPLETE,INS_RTKFIXED,37.37010082408,126.72084278410,9.8363,22.3000,-0.0077,0.0002,0.0002,-0.786930858,0.220983047,80.255496235,0.2109,0.1616,0.2842,0.0344,0.0343,0.0312,0.0727,0.0733,4.8905,0f000005,0*84218c18\n\tsystem status\tnormal 0 27.800000 0 0\trobot status\t0.680194\t-3.259887\t9.836300\t-0.786931\t0.220983\t9.744504\t0.000000\t0.000000\n\t\n15:54:50.1\tlog_raw\tgps_raw\t#INSPVAXA,USB3,0,53.0,FINESTEERING,2107,284104.050,02000000,471d,15824;INS_ALIGNMENT_COMPLETE,INS_RTKFIXED,37.37010082408,126.72084278410,9.8363,22.3000,-0.0077,0.0002,0.0002,-0.786930858,0.220983047,80.255496235,0.2109,0.1616,0.2842,0.0344,0.0343,0.0312,0.0727,0.0733,4.8905,0f000005,0*84218c18\n\tsystem status\tnormal 0 27.800000 0 0\trobot status\t0.680194\t-3.259887\t9.836300\t-0.786931\t0.220983\t9.744504\t0.000000\t0.000000\n\t\n15:54:50.6\tlog_raw\tgps_raw\t#INSPVAXA,USB3,0,53.0,FINESTEERING,2107,284104.050,02000000,471d,15824;INS_ALIGNMENT_COMPLETE,INS_RTKFIXED,37.37010082408,126.72084278410,9.8363,22.3000,-0.0077,0.0002,0.0002,-0.786930858,0.220983047,80.255496235,0.2109,0.1616,0.2842,0.0344,0.0343,0.0312,0.0727,0.0733,4.8905,0f000005,0*84218c18\n\tsystem status\tnormal 0 27.800000 0 0\trobot status\t0.680194\t-3.259887\t9.836300\t-0.786931\t0.220983\t9.744504\t0.000000\t0.000000\n\t\n15:54:51.1\tlog_raw\tgps_raw\t#INSPVAXA,USB3,0,53.0,FINESTEERING,2107,284104.050,02000000,471d,15824;INS_ALIGNMENT_COMPLETE,INS_RTKFIXED,37.37010082408,126.72084278410,9.8363,22.3000,-0.0077,0.0002,0.0002,-0.786930858,0.220983047,80.255496235,0.2109,0.1616,0.2842,0.0344,0.0343,0.0312,0.0727,0.0733,4.8905,0f000005,0*84218c18\n\tsystem status\tnormal 0 27.800000 0 0\trobot status\t0.680194\t-3.259887\t9.836300\t-0.786931\t0.220983\t9.744504\t0.000000\t0.000000\n\t\n15:54:51.6\tlog_raw\tgps_raw\t#INSPVAXA,USB3,0,53.0,FINESTEERING,2107,284104.050,02000000,471d,15824;INS_ALIGNMENT_COMPLETE,INS_RTKFIXED,37.37010082408,126.72084278410,9.8363,22.3000,-0.0077,0.0002,0.0002,-0.786930858,0.220983047,80.255496235,0.2109,0.1616,0.2842,0.0344,0.0343,0.0312,0.0727,0.0733,4.8905,0f000005,0*84218c18\n\tsystem status\tnormal 0 27.800000 0 0\trobot status\t0.680194\t-3.259887\t9.836300\t-0.786931\t0.220983\t9.744504\t0.000000\t0.000000\n\t\n15:54:52.1\tlog_raw\tgps_raw\t#INSPVAXA,USB3,0,53.0,FINESTEERING,2107,284104.050,02000000,471d,15824;INS_ALIGNMENT_COMPLETE,INS_RTKFIXED,37.37010082408,126.72084278410,9.8363,22.3000,-0.0077,0.0002,0.0002,-0.786930858,0.220983047,80.255496235,0.2109,0.1616,0.2842,0.0344,0.0343,0.0312,0.0727,0.0733,4.8905,0f000005,0*84218c18\n\tsystem status\tnormal 0 27.800000 0 0\trobot status\t0.680194\t-3.259887\t9.836300\t-0.786931\t0.220983\t9.744504\t0.000000\t0.000000\n\t\n15:54:52.6\tlog_raw\tgps_raw\t#INSPVAXA,USB3,0,53.0,FINESTEERING,2107,284104.050,02000000,471d,15824;INS_ALIGNMENT_COMPLETE,INS_RTKFIXED,37.37010082408,126.72084278410,9.8363,22.3000,-0.0077,0.0002,0.0002,-0.786930858,0.220983047,80.255496235,0.2109,0.1616,0.2842,0.0344,0.0343,0.0312,0.0727,0.0733,4.8905,0f000005,0*84218c18\n\tsystem status\tnormal 0 27.800000 0 0\trobot status\t0.680194\t-3.259887\t9.836300\t-0.786931\t0.220983\t9.744504\t0.000000\t0.000000\n\t\n15:54:53.1\tlog_raw\tgps_raw\t#INSPVAXA,USB3,0,53.0,FINESTEERING,2107,284104.050,02000000,471d,15824;INS_ALIGNMENT_COMPLETE,INS_RTKFIXED,37.37010082408,126.72084278410,9.8363,22.3000,-0.0077,0.0002,0.0002,-0.786930858,0.220983047,80.255496235,0.2109,0.1616,0.2842,0.0344,0.0343,0.0312,0.0727,0.0733,4.8905,0f000005,0*84218c18\n\tsystem status\tnormal 0 27.800000 0 0\trobot status\t0.680194\t-3.259887\t9.836300\t-0.786931\t0.220983\t9.744504\t0.000000\t0.000000\n\t\n15:54:53.6\tlog_raw\tgps_raw\t#INSPVAXA,USB3,0,53.0,FINESTEERING,2107,284104.050,02000000,471d,15824;INS_ALIGNMENT_COMPLETE,INS_RTKFIXED,37.37010082408,126.72084278410,9.8363,22.3000,-0.0077,0.0002,0.0002,-0.786930858,0.220983047,80.255496235,0.2109,0.1616,0.2842,0.0344,0.0343,0.0312,0.0727,0.0733,4.8905,0f000005,0*84218c18\n\tsystem status\tnormal 0 27.800000 0 0\trobot status\t0.680194\t-3.259887\t9.836300\t-0.786931\t0.220983\t9.744504\t0.000000\t0.000000\n\t\n15:54:54.1\tlog_raw\tgps_raw\t#INSPVAXA,USB3,0,53.0,FINESTEERING,2107,284104.050,02000000,471d,15824;INS_ALIGNMENT_COMPLETE,INS_RTKFIXED,37.37010082408,126.72084278410,9.8363,22.3000,-0.0077,0.0002,0.0002,-0.786930858,0.220983047,80.255496235,0.2109,0.1616,0.2842,0.0344,0.0343,0.0312,0.0727,0.0733,4.8905,0f000005,0*84218c18\n\tsystem status\tnormal 0 27.800000 0 0\trobot status\t0.680194\t-3.259887\t9.836300\t-0.786931\t0.220983\t9.744504\t0.000000\t0.000000\n\t\n15:54:54.6\tlog_raw\tgps_raw\t#INSPVAXA,USB3,0,53.0,FINESTEERING,2107,284104.050,02000000,471d,15824;INS_ALIGNMENT_COMPLETE,INS_RTKFIXED,37.37010082408,126.72084278410,9.8363,22.3000,-0.0077,0.0002,0.0002,-0.786930858,0.220983047,80.255496235,0.2109,0.1616,0.2842,0.0344,0.0343,0.0312,0.0727,0.0733,4.8905,0f000005,0*84218c18\n\tsystem 
